vi "GetCMYK.vi"(0 "ColorCMYK in":refnum<class "ColorCMYK.lvclass">, 11 "error in (no error)":errorcluster) -> (4 "ColorCMYK out":refnum<class "ColorCMYK.lvclass">, 6 "C (%)":dbl, 8 "M (%)":dbl, 10 "Y (%)":dbl, 14 "K (%)":dbl, 15 "error out":errorcluster)   [LabVIEW 2021, in "Picture2D.lvlib" / "ColorCMYK.lvclass"]
uses:
  ColorCMYK.lvclass
  ColorCMYK.lvclass/ColorCMYK.ctl
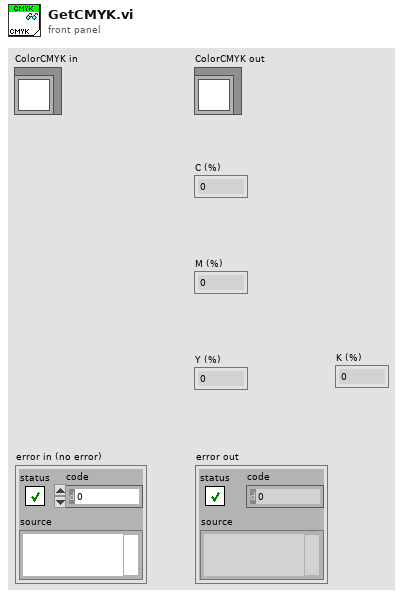
[diagram p1: front panel]
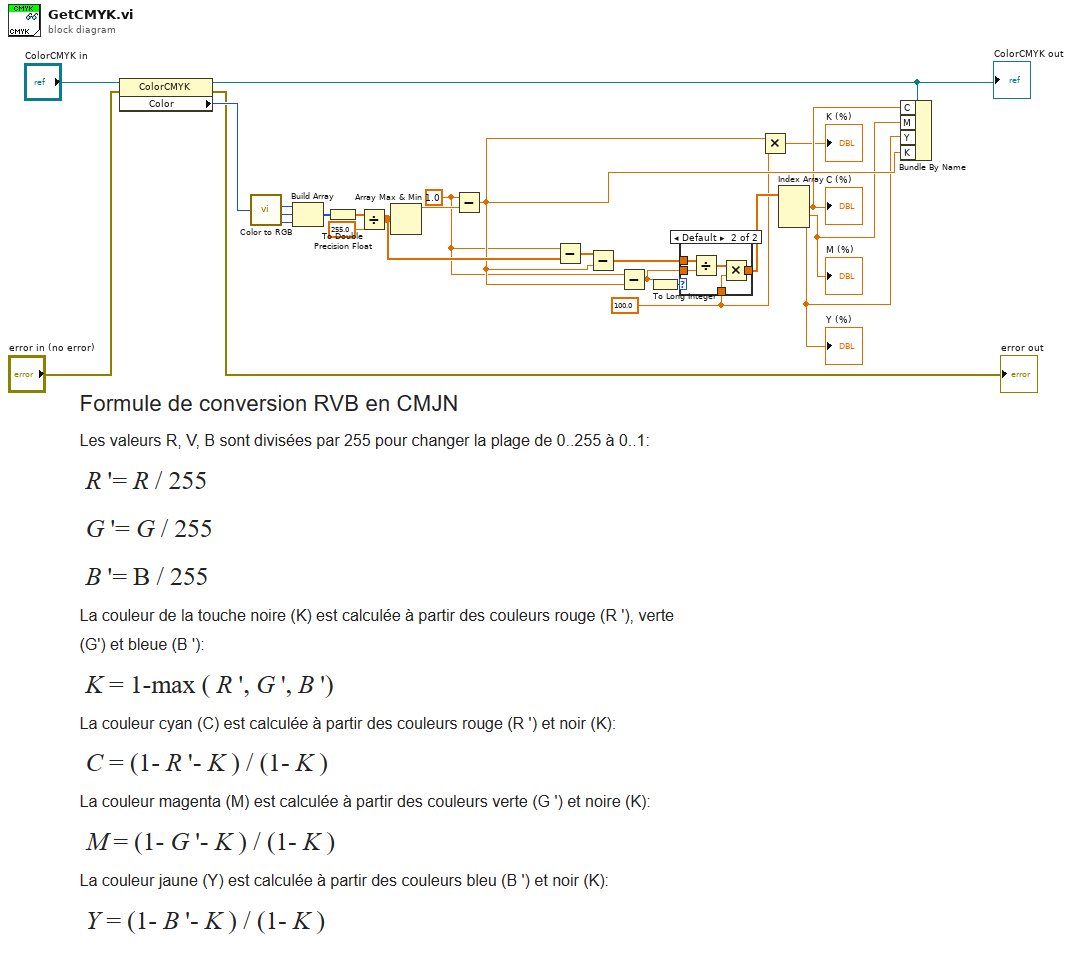
[diagram p0: block diagram]
diagram:
  w1 = 100.0
  w12 = 1.0 ("x")
  n1 = property class="ColorCMYK"(reference="ColorCMYK in", error in="error in (no error)") -> (reference out=w10:refnum<class "ColorCMYK.lvclass">, error out=→"error out":errorcluster, "Color"=w24:u32)
  "ColorCMYK out" <- w10
  n2 = call <vilib>:"Color to RGB.vi"("Color"=w24) -> ("R"=w23:u8, "G"=w22:u8, "B"=w21:u8)  [unwired: 1 out]
  n3 = Build Array(w23, w22, w21) -> (w20:u8[])
  n4 = To Double Precision Float(number=w20) -> (double precision float=w19:dbl[])
  n5 = Divide(x=w19, y=255.0) -> (x/y=w16:dbl[])
  n6 = Array Max & Min(array=w16) -> (max value=w17:dbl)  [unwired: 3 out]
  n7 = Subtract(x=w12, y=w17) -> (x-y=w14:dbl)
  n8 = Subtract(x=w12, y=w16) -> (x-y=w15:dbl[])
  n9 = Subtract(x=w15, y=w14) -> (x-y=w13:dbl[])
  n10 = Subtract(x=w12, y=w14) -> (x-y=w3:dbl)
  n11 = To Long Integer(number=w3) -> (32bit integer=w2:i32)
  n12 = case shown="Default" w2 {
    tunnel: w13 -> [_ w30]
    tunnel: w3 -> [_ w29]
    tunnel: [_ w27] -> w11
    tunnel: w1 -> [_ w26]
    frame 0 {
    }
    frame Default {
      n13 = Divide(x=w30, y=w29) -> (x/y=w28:dbl[])
      n14 = Multiply(x=w28, y=w26) -> (x*y=w27:dbl[])
    }
  }
  n15 = Multiply(x=w14, y=w1) -> (x*y=→"K (%)":dbl)
  n16 = Index Array(array=w11) -> (element #1=w9:dbl, element #2=w8:dbl, element #3=w7:dbl)  [unwired: 3 in]
  "C (%)" <- w9
  "M (%)" <- w8
  "Y (%)" <- w7
  n17 = Bundle By Name(cluster=w10, "C"=w9, "M"=w8, "Y"=w7, "K"=w14) -> ()  [unwired: 1 out]
